vi "ROS_Master_addPubSub.vi"(2 "PubSub":T1, 3 "ROS_Master in":T2) -> (1 "ROS_Master out":T2)   [LabVIEW 2015]
uses:
  ROS_Master.ctl
  ROS_Topic.ctl
  ROS_Node.ctl
  ROS_Service.ctl
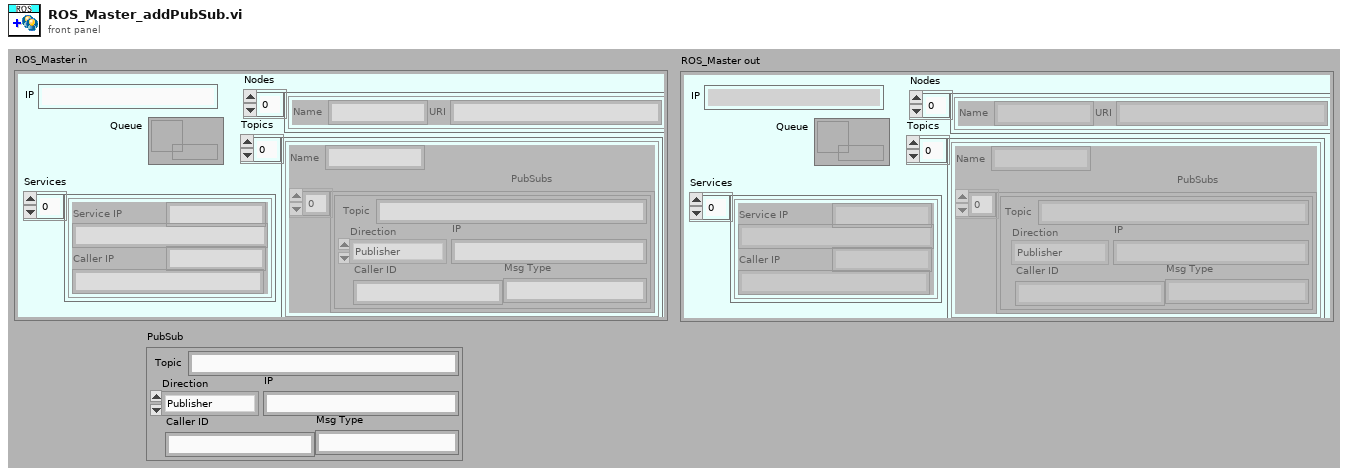
[diagram p1: front panel]
types:
  T1 = typedef "ROS_Topic.ctl" = cluster{"Caller ID":string, "IP":string, "Msg Type":string, "Direction":enum16{"Publisher", "Subscriber"}, "Topic":string}
  T2 = typedef "ROS_Master.ctl" = cluster{"IP":string, "Topics":cluster{"Name":string, "PubSubs":T1[]}[], "Nodes":T3[], "Services":T4[], "Queue":refnum<queue>}
  T3 = typedef "ROS_Node.ctl" = cluster{"Name":string, "URI":string}
  T4 = typedef "ROS_Service.ctl" = cluster{"Service":string, "Service IP":string, "Caller IP":string, "Caller ID":string}
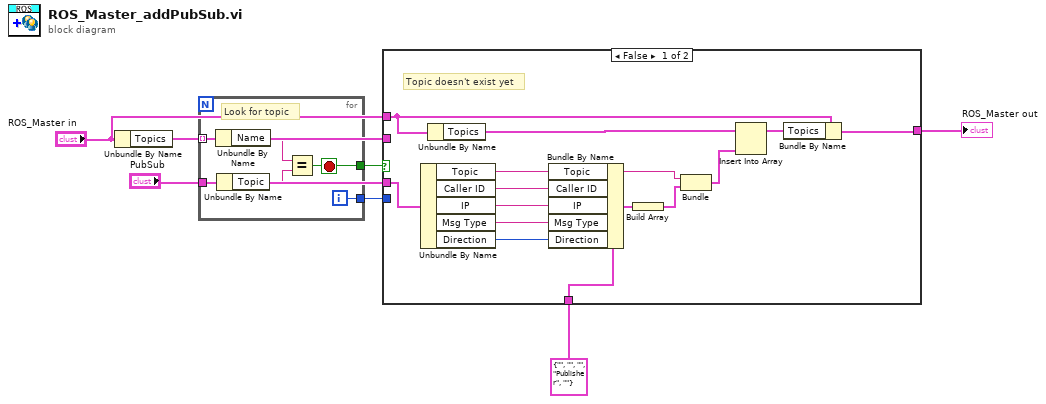
[diagram p0: block diagram]
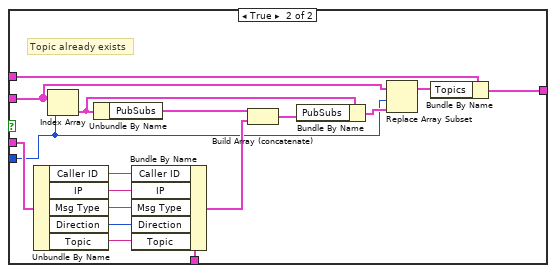
[diagram p2: hidden frame]
diagram:
  n1 = Unbundle By Name("ROS_Master in") -> ("Topics"=w5:cluster{"Name":string, "PubSubs":T1[]}[])
  n2 = for {
    tunnel: w5 -> [w13] mode=indexing
    tunnel: "PubSub" -> [w12]
    tunnel: [w9] -> w7
    tunnel: [w8] -> w6
    i -> [w8]
    stop <- w9 stop-if-true
    # "Look for topic"
    n3 = Unbundle By Name(w13) -> ("Name"=w11:string)
    n4 = Unbundle By Name(w12) -> ("Topic"=w10:string)
    n5 = Equal?(x=w11, y=w10) -> (x = y?=w9:bool)
  }
  n6 = case shown="False" w7 {
    tunnel: "PubSub" -> [w24 w44]
    tunnel: w6 -> [_ w32]
    tunnel: w5 -> [_ w36]
    tunnel: "ROS_Master in" -> [w19 w29]
    tunnel: [w17 w28] -> w3
    tunnel: T1 {"Caller ID"="", "IP"="", "Msg Type"="", "Direction"=enum."Publisher", "Topic"=""} ("PubSub") -> [w14 w33]
    frame False {
      # "Topic doesn't exist yet"
      n7 = Unbundle By Name(w24) -> ("Topic"=w15:string, "Caller ID"=w27:string, "IP"=w26:string, "Msg Type"=w25:string, "Direction"=w16:enum16{"Publisher", "Subscriber"})
      n8 = Unbundle By Name(w19) -> ("Topics"=w21:cluster{"Name":string, "PubSubs":T1[]}[])
      n9 = Bundle By Name(cluster=w14, "Topic"=w15, "Caller ID"=w27, "IP"=w26, "Msg Type"=w25, "Direction"=w16) -> (w23:T1)
      n10 = Build Array(w23) -> (w22:T1[])
      n11 = Bundle("Topic"=w15, w22) -> (w20:cluster{"Topic":string, T1[]})  [unwired: 1 in]
      n12 = Insert Into Array(array=w21, new element=w20) -> (w18:cluster{"Name":string, "PubSubs":T1[]}[])  [unwired: 1 in]
      n13 = Bundle By Name(cluster=w19, "Topics"=w18) -> (w17:T2)
    }
    frame True {
      # "Topic already exists"
      n14 = Unbundle By Name(w44) -> ("Caller ID"=w43:string, "IP"=w42:string, "Msg Type"=w41:string, "Direction"=w30:enum16{"Publisher", "Subscriber"}, "Topic"=w34:string)
      n15 = Index Array(array=w36, index=w32) -> (element=w39:cluster{"Name":string, "PubSubs":T1[]})
      n16 = Unbundle By Name(w39) -> ("PubSubs"=w31:T1[])
      n17 = Bundle By Name(cluster=w33, "Caller ID"=w43, "IP"=w42, "Msg Type"=w41, "Direction"=w30, "Topic"=w34) -> (w40:T1)
      n18 = Build Array (concatenate)(w31, w40) -> (w38:T1[])
      n19 = Bundle By Name(cluster=w39, "PubSubs"=w38) -> (w37:cluster{"Name":string, "PubSubs":T1[]})
      n20 = Replace Array Subset(array=w36, new element=w37, index=w32) -> (w35:cluster{"Name":string, "PubSubs":T1[]}[])
      n21 = Bundle By Name(cluster=w29, "Topics"=w35) -> (w28:T2)
    }
  }
  "ROS_Master out" <- w3
